vi "ABB Report paging.vi"(9 "String":string) -> (0 "page ends":i32[](array[numeric]), 1 "result string":string, 2 "Page Names":string[](array[string]), 3 "Total pages":i32)   [LabVIEW 2017]
uses:
  ABB global.vi
panel:
  out "end":i32
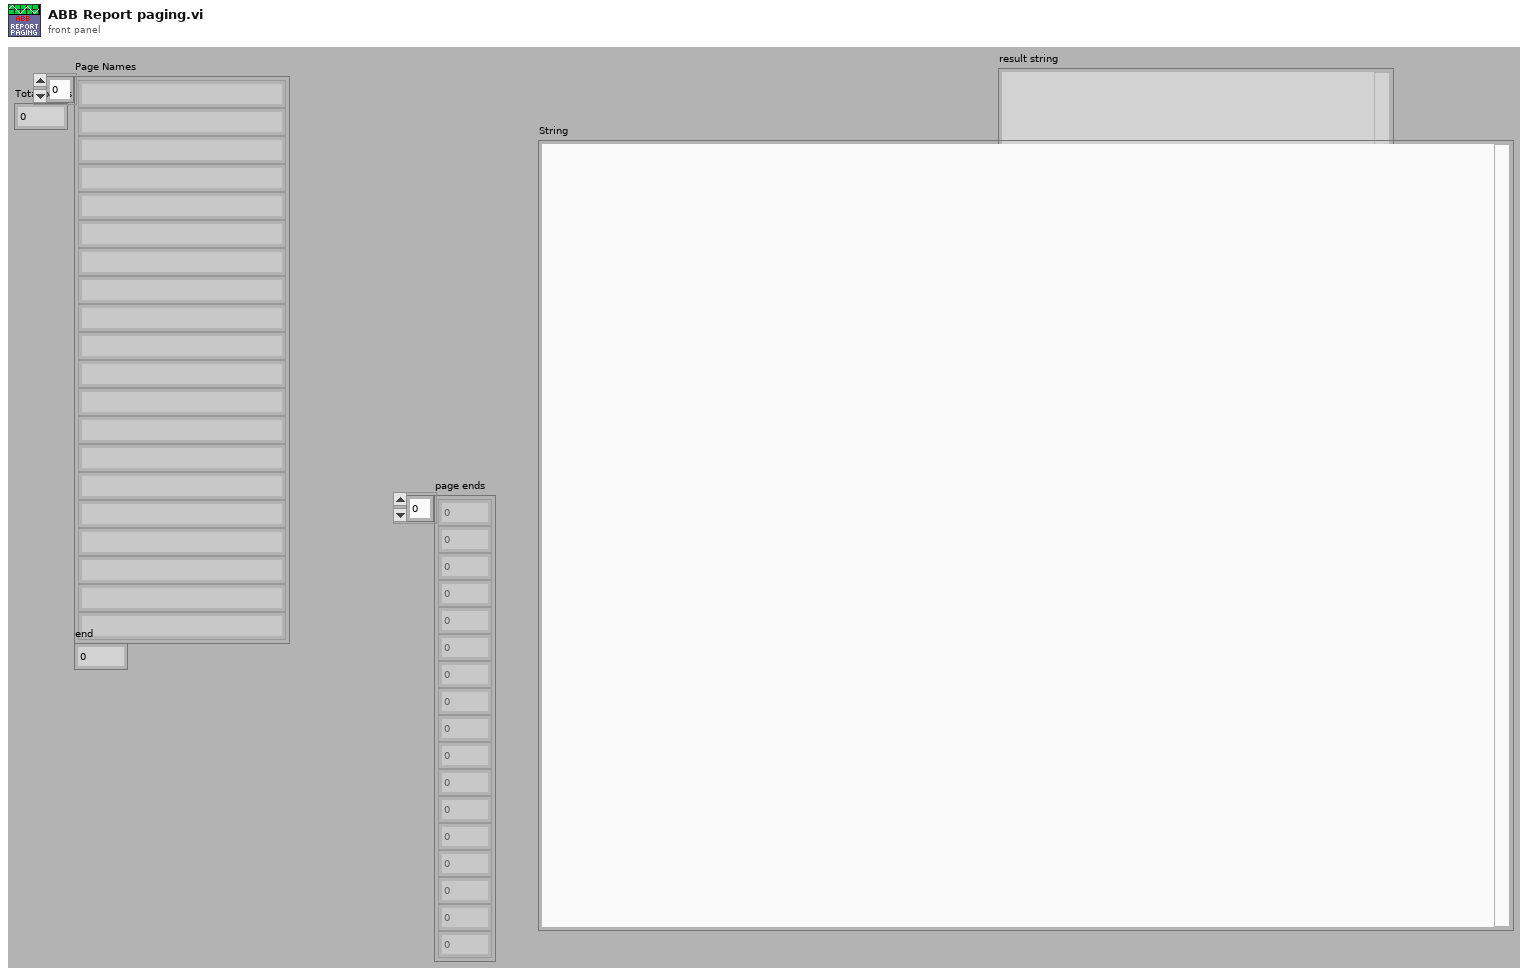
[diagram p1: front panel]
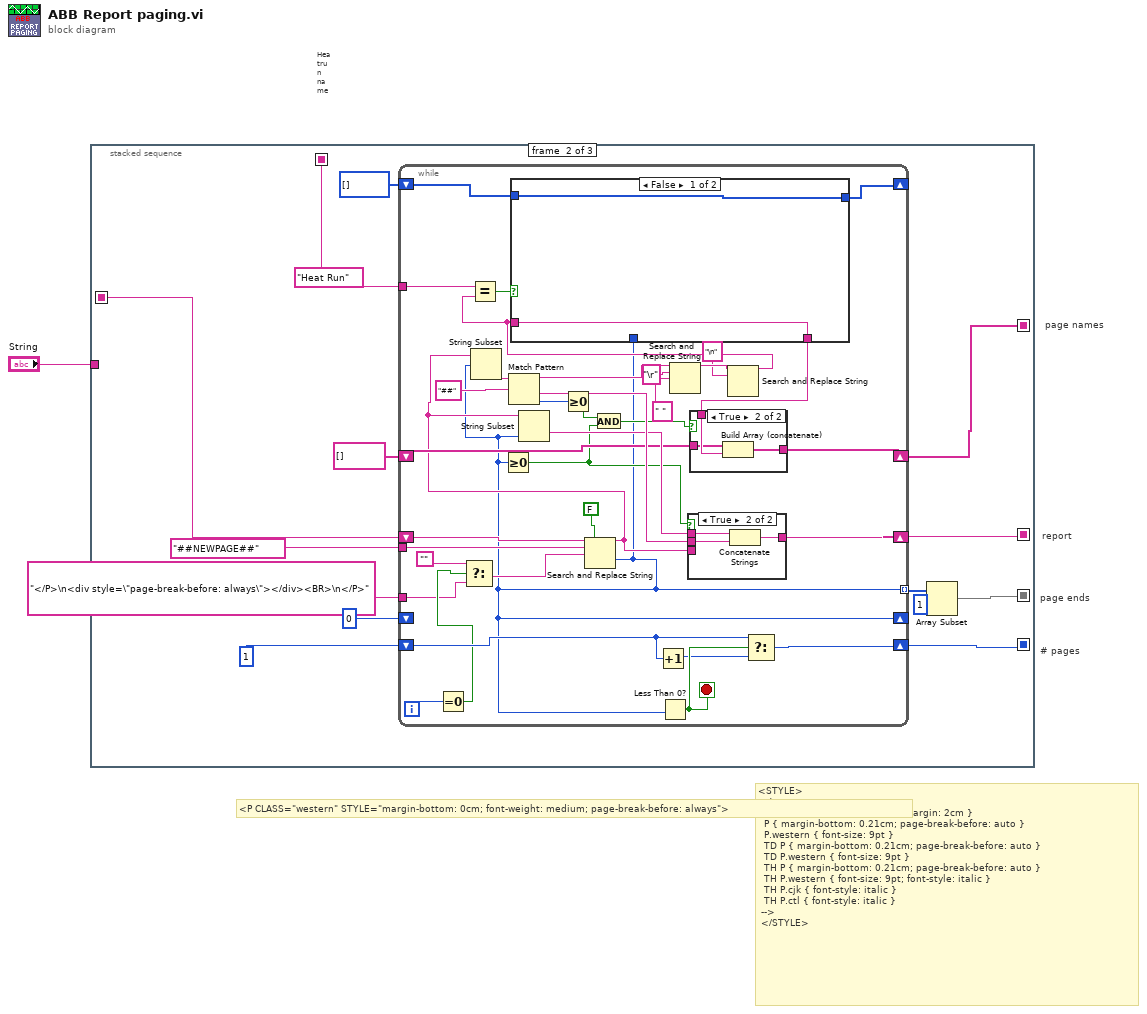
[diagram p0: block diagram]
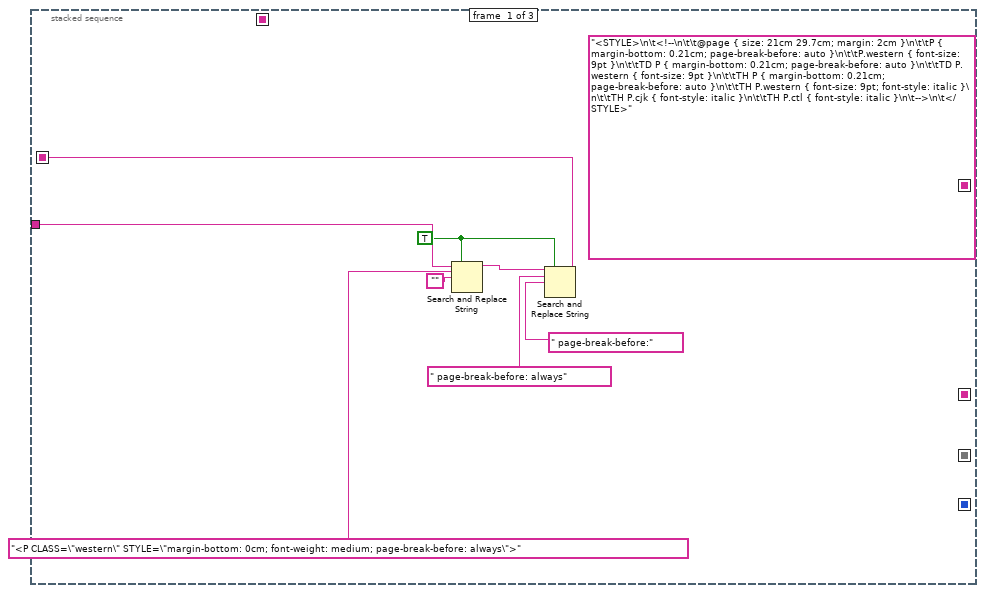
[diagram p2: hidden frame]
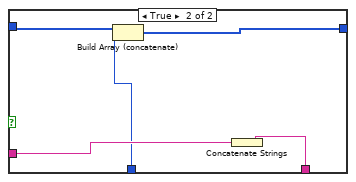
[diagram p3: hidden frame]
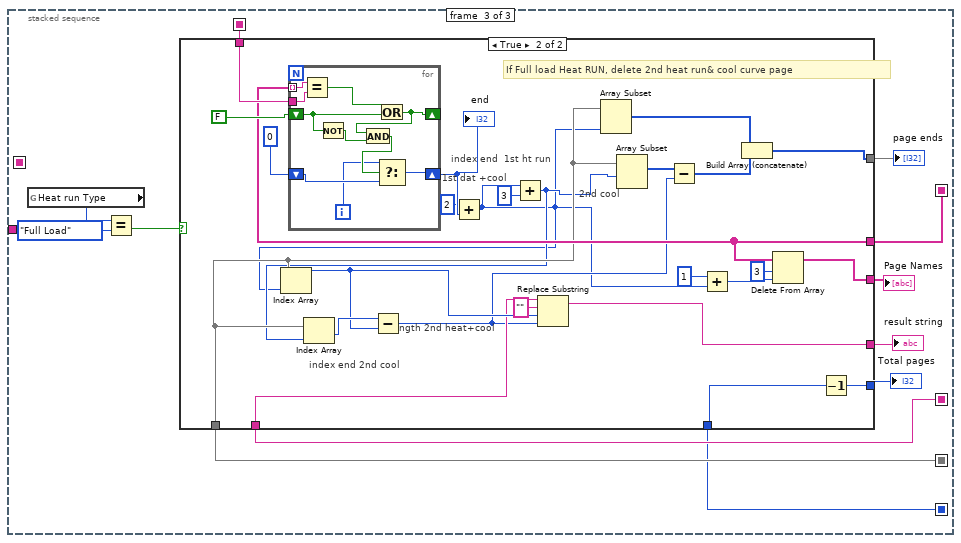
[diagram p6: hidden frame]
diagram:
  # "Heatrun name"
  # "page names"
  # "# pages"
  # "page ends"
  # "report"
  # "<STYLE>\n\t<!--\n\t\t@page { size: 21cm 29.7cm; margin: 2cm }\n\t\tP { margin-bottom: 0.21cm; page-break-before: auto }\n\t\tP.western { font-size: 9pt }\n\t\tTD P { margin-bottom: 0.21cm; page-break-before: auto }\n\t\tTD P.western { font-size: 9pt }\n\t\tTH P { margin-bottom: 0.21cm; page-break-before: auto }\n\t\tTH P.western { font-size: 9pt; font-style: italic }\n\t\tTH P.cjk { font-style: italic }\n\t\tTH P.ctl { font-style: italic }\n\t-->\n\t</STYLE>"
  # "<P CLASS=\"western\" STYLE=\"margin-bottom: 0cm; font-weight: medium; page-break-before: always\">"
  n1 = stacked-sequence {
    seq-local: [w5 _ _] -> [_ w17 _]
    seq-local: [_ w14 _] -> [_ _ w86]
    seq-local: [_ w13 _] -> [_ _ w81]
    seq-local: [_ w12 _] -> [_ _ w85]
    seq-local: [_ w11 _] -> [_ _ w84]
    seq-local: [_ w10 _] -> [_ _ w80]
    tunnel: "String" -> [w9 _ _]
    frame #0 {
      w2 = TRUE ("replace all? (F)")
      (unwired) "<STYLE>\n\t<!--\n\t\t@page { size: 21cm 29.7cm; margin: 2cm }\n\t\tP { margin-bottom: 0.21cm; page-break-before: auto }\n\t\tP.western { font-size: 9pt }\n\t\tTD P { margin-bottom: 0.21cm; page-break-before: auto }\n\t\tTD P.western { font-size: 9pt }\n\t\tTH P { margin-bottom: 0.21cm; page-break-before: auto }\n\t\tTH P.western { font-size: 9pt; font-style: italic }\n\t\tTH P.cjk { font-style: italic }\n\t\tTH P.ctl { font-style: italic }\n\t-->\n\t</STYLE>"
      n2 = Search and Replace String(replace all?=w2, input string=w9, search string="<P CLASS=\"western\" STYLE=\"margin-bottom: 0cm; font-weight: medium; page-break-before: always\">", replace string="" ("replace string (\"\")")) -> (result string=w6:string)  [unwired: 4 in, 3 out]
      n3 = Search and Replace String(replace all?=w2, input string=w6, search string=" page-break-before: always", replace string=" page-break-before:") -> (result string=w5:string)  [unwired: 4 in, 3 out]
    }
    frame #1 {
      w12 = "Heat Run" ("x")
      n4 = while {
        tunnel: "</P>\n<div style=\"page-break-before: always\"></div><BR>\n</P>" ("replace string (\"\")") -> [w33]
        tunnel: "##NEWPAGE##" ("search string") -> [w34]
        shift-right: [w52] -> w13
        shift-left: w17 -> [w38]
        shift-right: [w57] -> w10
        shift-left: 1 -> [w55]
        shift-right: [w25] -> _
        shift-left: 0 ("offset past replacement") -> [_]
        tunnel: [w25] -> w20 mode=indexing
        shift-right: [w26] -> w14
        shift-left: string[] [] -> [w41]
        shift-right: [w30] -> _
        shift-left: i32[] [] -> [w27]
        tunnel: w12 -> [w24]
        i -> [w37]
        stop <- w58 stop-if-true
        n5 = Equal To 0?(x=w37) -> (x = 0?=w36:bool)
        n6 = Select(t="", s=w36, f=w33) -> (s? t:f=w32:string)
        n7 = Search and Replace String(replace all?=FALSE ("replace all? (F)"), input string=w38, search string=w34, replace string=w32) -> (result string=w39:string, offset past replacement=w25:i32)  [unwired: 4 in, 2 out]
        n8 = String Subset(string=w39, offset (0)=w25) -> (substring=w50:string)  [unwired: 1 in]
        n9 = Greater Or Equal To 0?(x=w25) -> (x >= 0?=w40:bool)
        n10 = Match Pattern(string=w50, regular expression="##") -> (before substring=w49:string, after substring=w53:string, offset past match=w44:i32)  [unwired: 1 in, 1 out]
        n11 = String Subset(string=w39, length (rest)=w25) -> (substring=w51:string)  [unwired: 1 in]
        n12 = Greater Or Equal To 0?(x=w44) -> (x >= 0?=w43:bool)
        n13 = And(x=w43, y=w40) -> (x .and. y?=w42:bool)
        n14 = Increment(x=w55) -> (x+1=w56:i32)
        n15 = Less Than 0?(x=w25) -> (x < 0?=w58:bool)
        n16 = Search and Replace String(input string=w49, search string="\r", replace string=" " ("search string")) -> (result string=w46:string)  [unwired: 5 in, 3 out]
        n17 = case shown="True" w40 {
          tunnel: w53 -> [_ w70]
          tunnel: [w67 w69] -> w52
          tunnel: w51 -> [_ w68]
          tunnel: w39 -> [w67 _]
          frame False {
          }
          frame True {
            n18 = Concatenate Strings(w68, w70) -> (w69:string)
          }
        }
        n19 = Search and Replace String(input string=w46, search string="\n") -> (result string=w29:string)  [unwired: 6 in, 3 out]
        n20 = Equal?(x=w24, y=w29) -> (x = y?=w31:bool)
        n21 = case shown="False" w31 {
          tunnel: w27 -> [w61 w63]
          tunnel: [w61 w66] -> w30
          tunnel: w29 -> [w60 w65]
          tunnel: [w60 w64] -> w28
          tunnel: w25 -> [_ w62]
          frame False {
          }
          frame True {
            n22 = Build Array (concatenate)(w63, w62) -> (w66:i32[])
            n23 = Concatenate Strings(w65) -> (w64:string)
          }
        }
        n24 = case shown="True" w42 {
          tunnel: w28 -> [_ w74]
          tunnel: w41 -> [w71 w73]
          tunnel: [w71 w72] -> w26
          frame False {
          }
          frame True {
            n25 = Build Array (concatenate)(w73, w74) -> (w72:string[])
          }
        }
        n26 = Select(t=w55, s=w58, f=w56) -> (s? t:f=w57:i32)
      }
      n27 = Array Subset(array=w20, index=1) -> (w11:i32[])  [unwired: 1 in]
    }
    frame #2 {
      n28 = global read "ABB global.vi" "Heat run Type"() -> (w83:enum16{"Full Load", "Partial- & No-Load"})
      n29 = Equal?(x=w83, y=enum16{"Full Load", "Partial Load"}."Full Load") -> (x = y?=w75:bool)
      n30 = case shown="True" w75 {
        tunnel: w86 -> [w89 w106]
        tunnel: w85 -> [_ w116]
        tunnel: w84 -> [w87 w103]
        tunnel: w81 -> [w90 w108]
        tunnel: w80 -> [w88 w112]
        tunnel: [w90 w107] -> w79
        tunnel: [w89 w105] -> w78
        tunnel: [w88 w113] -> w77
        tunnel: [w87 w98] -> w76
        frame False {
        }
        frame True {
          # "2nd cool"
          # "1st dat +cool"
          # "index end 2nd cool"
          # "length 2nd heat+cool"
          # "index end  1st ht run"
          # "If Full load Heat RUN, delete 2nd heat run& cool curve page"
          n31 = for {
            tunnel: w106 -> [w126] mode=indexing
            tunnel: w116 -> [w124]
            shift-right: [w121] -> _
            shift-left: FALSE -> [w123]
            shift-right: [w118] -> w97
            shift-left: 0 ("offset past replacement") -> [w119]
            i -> [w117]
            n32 = Equal?(x=w126, y=w124) -> (x = y?=w125:bool)
            n33 = Not(x=w123) -> (.not. x?=w122:bool)
            n34 = Or(x=w125, y=w123) -> (x .or. y?=w121:bool)
            n35 = And(x=w121, y=w122) -> (x .and. y?=w120:bool)
            n36 = Select(t=w117, s=w120, f=w119) -> (s? t:f=w118:i32)
          }
          "end" <- w97
          n37 = Add(x=2, y=w97) -> (x+y=w94:i32)
          n38 = Index Array(array=w103, index=w94) -> (element=w110:i32)
          n39 = Add(x=w94, y=3) -> (x+y=w95:i32)
          n40 = Index Array(array=w103, index=w95) -> (element=w111:i32)
          n41 = Subtract(x=w111, y=w110) -> (x-y=w101:i32)
          n42 = Replace Substring(2:w101, 3:w110, 4:"" ("substring (\"\")"), 5:w108) -> (1:w107:string)  [unwired: 1 out]
          n43 = Array Subset(array=w103, length=w94) -> (w100:i32[])  [unwired: 1 in]
          n44 = Array Subset(array=w103, index=w95) -> (w102:i32[])  [unwired: 1 in]
          n45 = Subtract(x=w102, y=w101) -> (x-y=w99:i32[])
          n46 = Add(x=1, y=w94) -> (x+y=w93:i32)
          n47 = Build Array (concatenate)(w100, w99) -> (w98:i32[])
          n48 = Delete From Array "Delete From Array"(array=w106, length=3, index=w93) -> (array with subset deleted=w105:string[])  [unwired: 1 out]
          n49 = Decrement(x=w112) -> (x-1=w113:i32)
        }
      }
      "result string" <- w79
      "Page Names" <- w78
      "Total pages" <- w77
      "page ends" <- w76
    }
  }
